vi "Error Converter (ErrCode or Status).vi"(8 "error in (no error)":errorcluster, 11 "error code":i32) -> (0 "error out":errorcluster)   [LabVIEW 2020, in "NI_WebServices.lvlib"]
uses:
  <vilib>/wsapi/NI_WebServices.lvlib
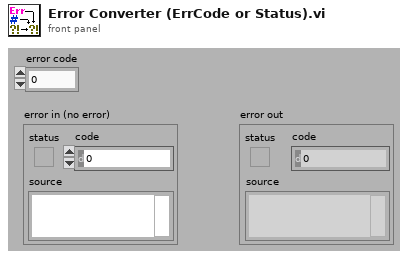
[diagram p1: front panel]
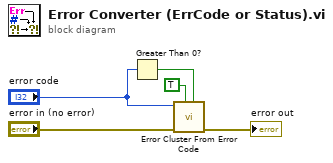
[diagram p0: block diagram]
diagram:
  n1 = Greater Than 0?(x="error code") -> (x > 0?=w1:bool)
  n2 = call <vilib>:"Error Cluster From Error Code.vi"("is warning? (False)"=w1, "show call chain? (False)"=TRUE, "error in (no error)"="error in (no error)", "error code (0)"="error code") -> ("error out"=→"error out":errorcluster)  [unwired: 5 in]
